vi "B field arrays.vi"() -> ()   [LabVIEW 2016]
panel:
  out "Waveform Graph 2":dbl[][](graph)
  out "Waveform Graph":i32[][](graph)=[[122, 457], [122, 457], [122, 457], [122, 457], [120, 457], [121, 457], [120, 457], [121, 457], [120, 457], [121, 457], [121, 457], [121, 457], [121, 457], [121, 457], [120, 457], [121, 457], [120, 457], [121, 457], [121, 457], [121, 457], [121, 457], [121, 457], [120, 457], [121, 457], [121, 457], [121, 457], [121, 457], [121, 457], [121, 457], [121, 457], [121, 457], [121, 457], [121, 457], [121, 457], [120, 457], [121, 457], [121, 457], [121, 457]]
  in  "B fields":dbl[][](array[numeric])=array38x122[4636 elements]
  in  "Array":i32[][](array[numeric])=[[122, 457], [122, 457], [122, 457], [122, 457], [120, 457], [121, 457], [120, 457], [121, 457], [120, 457], [121, 457], [121, 457], [121, 457], [121, 457], [121, 457], [120, 457], [121, 457], [120, 457], [121, 457], [121, 457], [121, 457], [121, 457], [121, 457], [120, 457], [121, 457], [121, 457], [121, 457], [121, 457], [121, 457], [121, 457], [121, 457], [121, 457], [121, 457], [121, 457], [121, 457], [120, 457], [121, 457], [121, 457], [121, 457]]
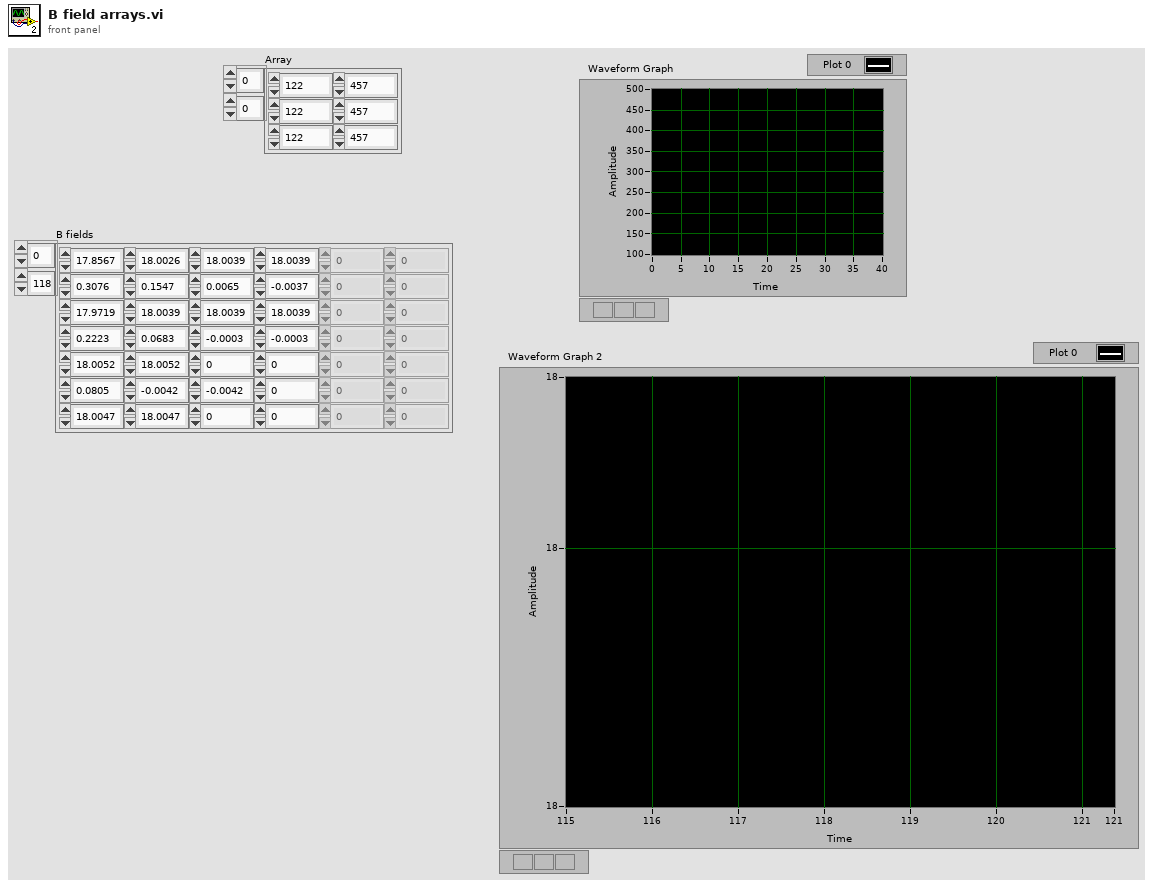
[diagram p1: front panel]
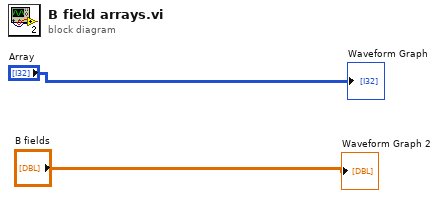
[diagram p0: block diagram]
diagram:
  "Waveform Graph" <- "Array"
  "Waveform Graph 2" <- "B fields"
